vi "generate_analogue_out_waveform.vi"(6 "sampling info":cluster{"Fs":dbl, "#s":dbl}={"Fs"=1000.0, "#s"=1000.0} {"Fs" format="%.2p"}, 7 "Reset signal":bool, 8 "error in (no error)":errorcluster, 9 "Camera start trigger phase":dbl, 10 "Vetl sine":T1, 11 "Vgalvo sine":T1) -> (0 "error out":errorcluster, 1 "Waveform Graph":waveform(dbl)[](graph))   [LabVIEW 2017]
uses:
  <vilib>/measure/NI_MABase.lvlib
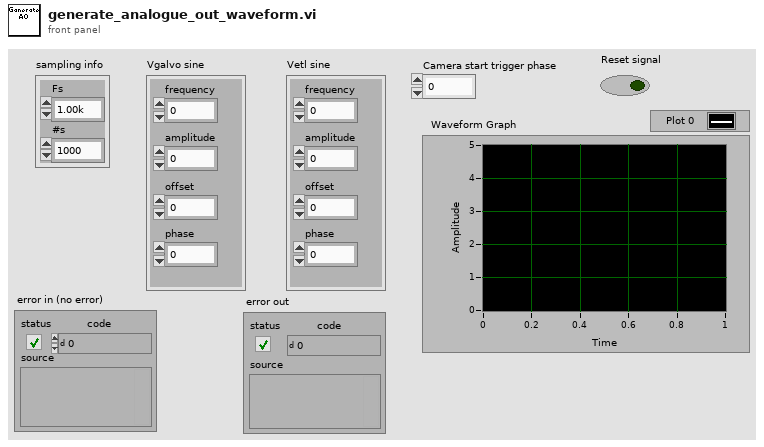
[diagram p1: front panel]
types:
  T1 = cluster{"frequency":dbl, "amplitude":dbl, "offset":dbl, "phase":dbl}
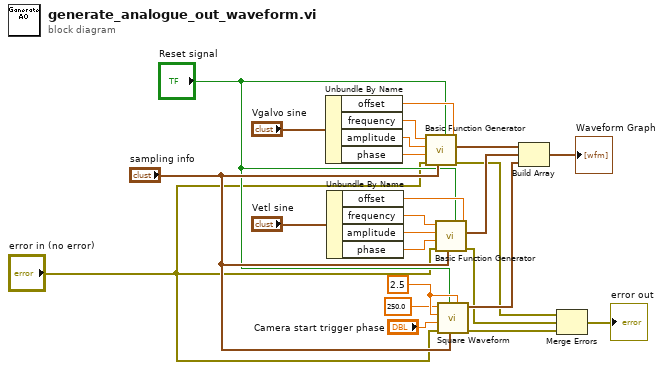
[diagram p0: block diagram]
diagram:
  w21 = 2.5
  n1 = Unbundle By Name("Vgalvo sine") -> ("offset"=w13:dbl, "frequency"=w16:dbl, "amplitude"=w15:dbl, "phase"=w14:dbl)
  n2 = Unbundle By Name("Vetl sine") -> ("offset"=w12:dbl, "frequency"=w9:dbl, "amplitude"=w10:dbl, "phase"=w11:dbl)
  n3 = call <vilib>:"Basic Function Generator.vi"("offset"=w13, "reset signal"="Reset signal", "sampling info"="sampling info", "error in (no error)"="error in (no error)", "phase"=w14, "amplitude"=w15, "frequency"=w16) -> ("error out"=w4:errorcluster, "signal out"=w23:waveform(dbl))  [unwired: 2 in, 1 out]
  n4 = call <vilib>:"Basic Function Generator.vi"("offset"=w12, "reset signal"="Reset signal", "sampling info"="sampling info", "error in (no error)"="error in (no error)", "phase"=w11, "amplitude"=w10, "frequency"=w9) -> ("error out"=w3:errorcluster, "signal out"=w24:waveform(dbl))  [unwired: 2 in, 1 out]
  n5 = call <vilib>:"Square Waveform.vi"("offset"=w21, "sampling info"="sampling info", "reset signal"="Reset signal", "error in (no error)"="error in (no error)", "phase"="Camera start trigger phase", "amplitude"=w21, "frequency"=250.0) -> ("error out"=w2:errorcluster, "signal out"=w22:waveform(dbl))  [unwired: 3 in]
  n6 = Build Array(w23, w24, w22) -> (→"Waveform Graph":waveform(dbl)[])
  n7 = Merge Errors(w4, w3, w2) -> (→"error out":errorcluster)
